vi "Read from File.vi"(8 "error in (no error)":errorcluster, 11 "Macro in":refnum<class "Macro.lvclass">) -> (0 "error out":errorcluster, 3 "Macro out":refnum<class "Macro.lvclass">)   [LabVIEW 2020, in "MacroAssert.lvlib" / "Macro.lvclass"]
uses:
  Macro.lvclass
  Macro.lvclass/Macro.ctl
  <vilib>/Utility/config.llb/NI_LVConfig.lvlib
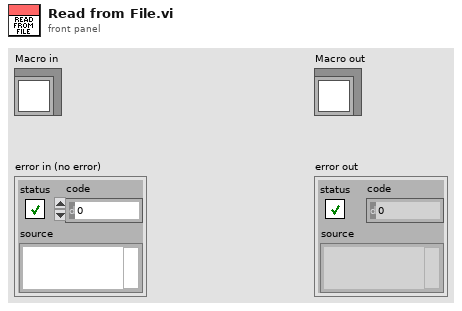
[diagram p1: front panel]
types:
  T1 = typedef "NI_LVConfig.lvlib/Config Data RefNum.ctl" = refnum<k1>
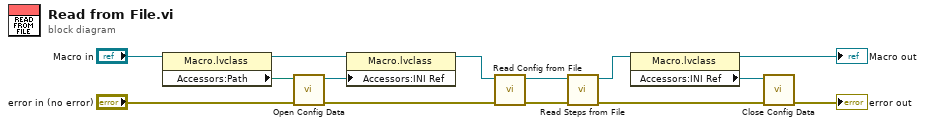
[diagram p0: block diagram]
diagram:
  n1 = property class="Macro.lvclass"(reference="Macro in") -> (reference out=w11:refnum<class "Macro.lvclass">, "Accessors:Path"=w12:path)  [unwired: 1 in, 1 out]
  n2 = call <vilib>:"Open Config Data.vi"("error in (no error)"="error in (no error)", "configuration file path"=w12) -> ("error out"=w9:errorcluster, "refnum"=w10:T1)  [unwired: 7 in, 1 out]
  n3 = property class="Macro.lvclass"(reference=w11, "Accessors:INI Ref"=w10) -> (reference out=w7:refnum<class "Macro.lvclass">)  [unwired: 1 in, 1 out]
  n4 = call-dynamic "Read Config from File.vi"("error in (no error)"=w9, "Macro in"=w7) -> ("error out"=w6:errorcluster, "Macro out"=w8:refnum<class "Macro.lvclass">)  [unwired: 8 in]
  n5 = call-dynamic "Read Steps from File.vi"("error in (no error)"=w6, "Macro in"=w8) -> ("error out"=w4:errorcluster, "Macro out"=w5:refnum<class "Macro.lvclass">)  [unwired: 8 in]
  n6 = property class="Macro.lvclass"(reference=w5) -> (reference out=→"Macro out":refnum<class "Macro.lvclass">, "Accessors:INI Ref"=w3:T1)  [unwired: 1 in, 1 out]
  n7 = call <vilib>:"Close Config Data.vi"("error in (no error)"=w4, "refnum"=w3) -> ("error out"=→"error out":errorcluster)  [unwired: 8 in, 1 out]
